vi "Read EndOfFile.vi"(8 "error in (no error)":errorcluster, 11 "ExistingFileMgr in":refnum<class "ExistingFileMgr.lvclass">) -> (0 "error out":errorcluster, 2 "EndOfFile":bool, 3 "ExistingFileMgr out":refnum<class "ExistingFileMgr.lvclass">)   [LabVIEW 2019, in "ExistingFileMgr.lvclass"]
uses:
  ExistingFileMgr.lvclass
  ExistingFileMgr.lvclass/ExistingFileMgr.ctl
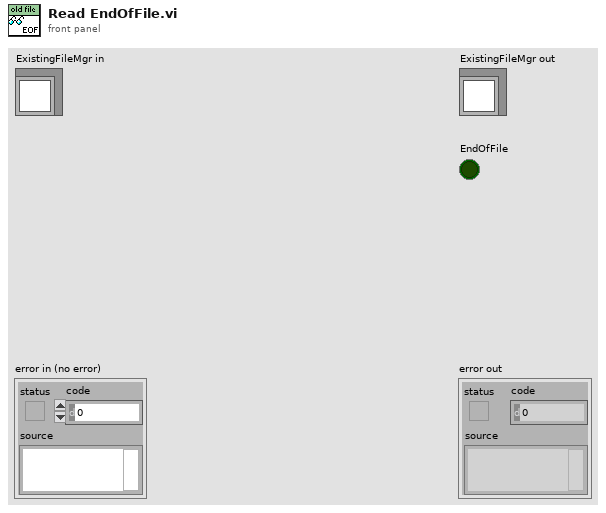
[diagram p1: front panel]
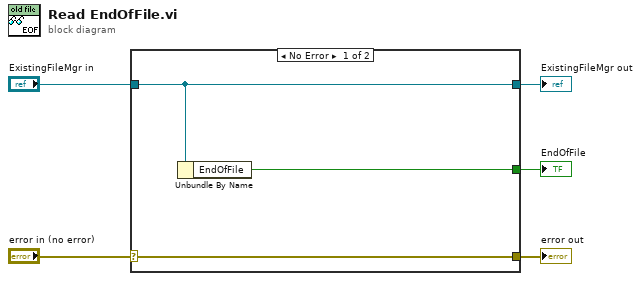
[diagram p0: block diagram]
diagram:
  n1 = case shown="No Error" "error in (no error)" {
    selector: "error in (no error)" -> [w8 w9]
    tunnel: [w8 w9] -> w4
    tunnel: [w7 w10] -> w2
    tunnel: "ExistingFileMgr in" -> [w7 w10]
    tunnel: [w6 _] -> w1
    frame No Error {
      n2 = Unbundle By Name(w7) -> ("EndOfFile"=w6:bool)
    }
    frame Error {
    }
  }
  "error out" <- w4
  "ExistingFileMgr out" <- w2
  "EndOfFile" <- w1
